vi "MotorControl.vi"() -> ()   [LabVIEW 2017]
panel:
  out "output cluster":T1={"Motor Relative"=[0.0, 0.0, 0.0, 0.0], "Motor absolute"=[0.0, 0.0, 0.0, 0.0], "Motor zero"=[0.0, 0.0, 0.0, 0.0], "Time between steps"=0.0, "Conversion (steps/mm)"=[31496.063, 31496.063, 31496.063, 12500.0], "Distance  (mm)"=[-100.0, 0.0, 0.0, 0.0], "run number"=37, "Number of steps"=1}
  in  "Module?":bool=TRUE
  in  "Stop":bool
  in  "Motor control":enum32{"Movement", "Setup", "Error"}(tab)
  in  "Single motion":bool=TRUE
  out "Step number":i32=1
  out "Motor Relative":dbl[](array[numeric])
  in  "Speed (mm/s)":dbl[](array[numeric])=[10.0, 1.0, 5.0, 10.0] format="%#_13g"
  in  "Distance  (mm)":dbl[](array[numeric])=[-100.0, 0.0, 0.0, 0.0] format="%#_13g"
  in  "Send":bool
  in  "Stop motion":bool
  out "Moving":bool
  out "Acquiring":bool
  in  "Go to zero":bool
  out "Motor Status":bool=TRUE
  out "Number of steps":i32=1
  out "Time between steps":dbl format="%#_13g"
  out "run number":i32=37
  in  "Reset motor":bool
  in  "Inc run #":bool
  in  "Zero C":bool
  in  "Zero B":bool
  in  "Zero A":bool
  in  "Zero D":bool
  in  "Motor zero":dbl[](array[numeric])=[0.0, 0.0, 0.0, 0.0] format="%#_13g"
  out "Motor absolute":dbl[](array[numeric])
  in  "Motor Port":string="COM12 19200"
  in  "Time between steps ctrl":dbl=5.0 caption="Time Target (s)"
  in  "# steps ctrl":i32=3
  in  "Conversion (steps/mm)":dbl[](array[numeric])=[31496.063, 31496.063, 31496.063, 12500.0] format="%#_13g"
  in  "Reset distance after run":bool
  in  "auto inc run #":bool
  out "error out":errorcluster={"status"=TRUE, "code"=-2147467259, "source"="Exception occured in Galil: 5001 OPEN ERROR.  OFFLINE specified to Galil::Galil()\n in MotorControl.vi"}
  out "Library Version":string="GalilClass1.dll 1.5.0.0\r\nGalil1.dll 1.6.4.580"
  out "Connect To:":string="COM12 19200, DMC2182sH2a, 16295"
  in  "Galil.IGalil":refnum<k7>
  # "spend time updating output cluster?"
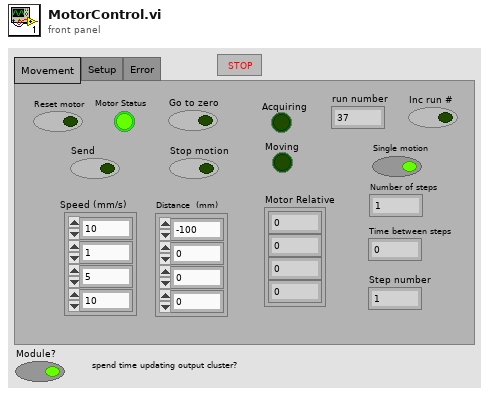
[diagram p1: front panel]
types:
  T1 = cluster{"Motor Relative":dbl[], "Motor absolute":dbl[], "Motor zero":dbl[], "Time between steps":dbl, "Conversion (steps/mm)":dbl[], "Distance  (mm)":dbl[], "run number":i32, "Number of steps":i32}
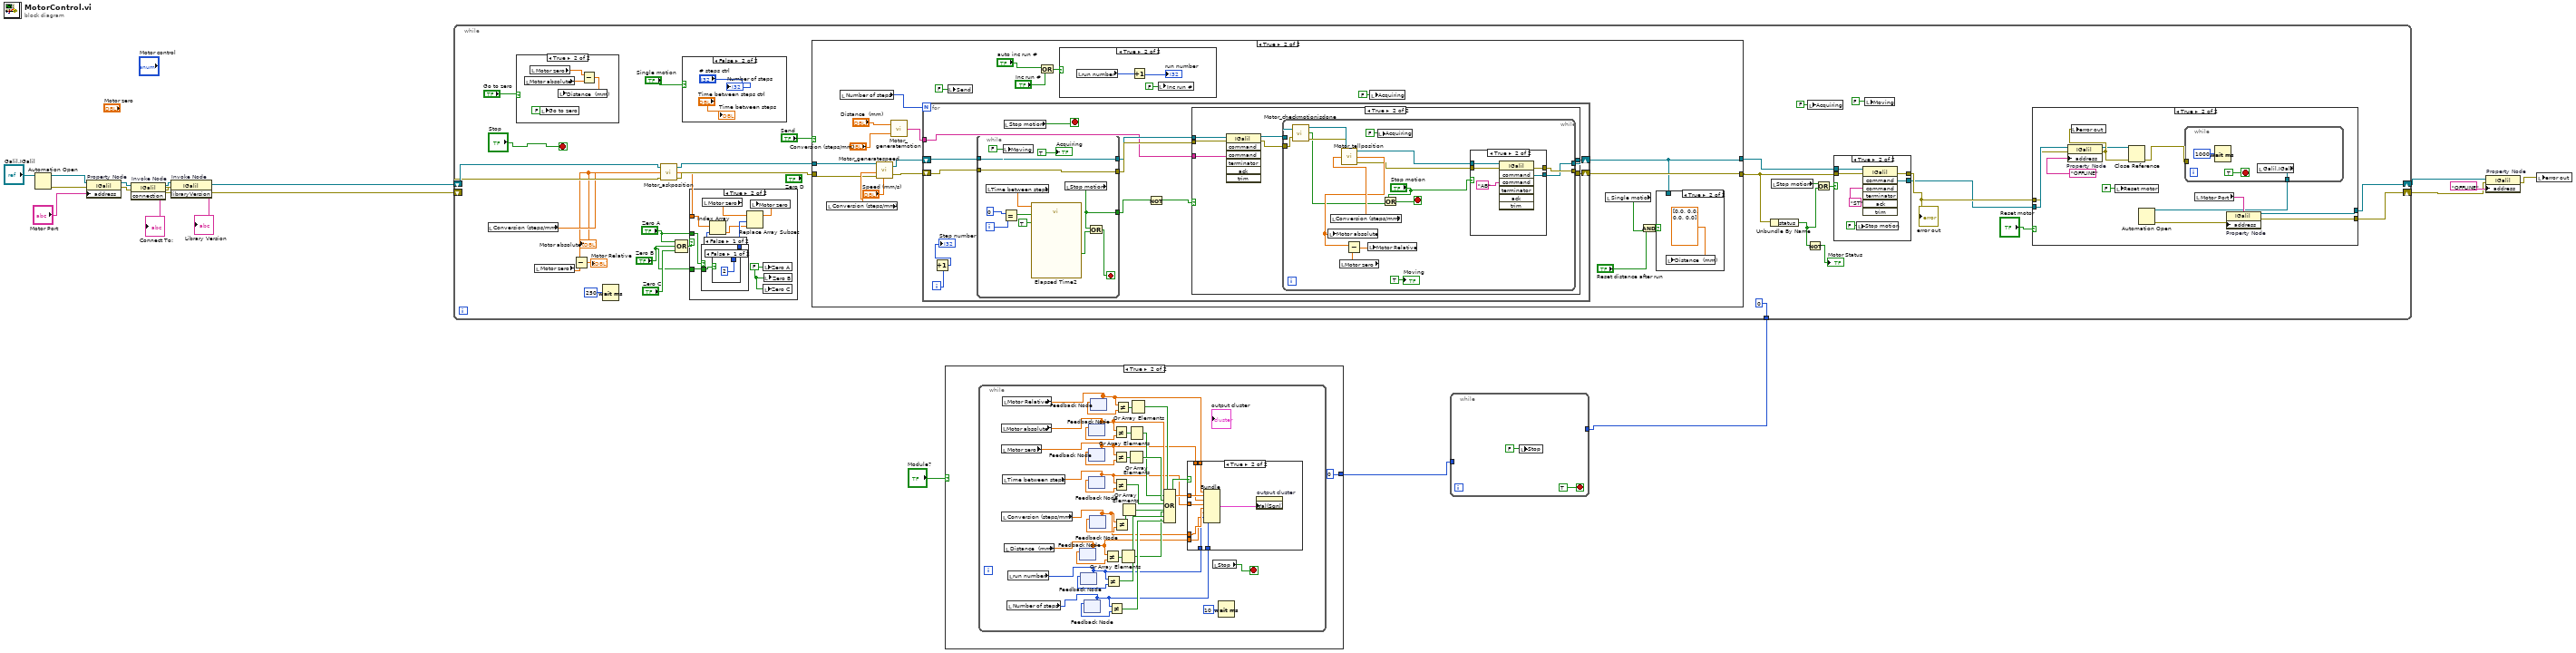
[diagram p0: block diagram]
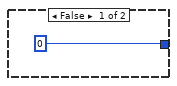
[diagram p2: hidden frame]
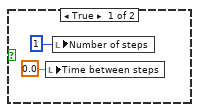
[diagram p7: hidden frame]
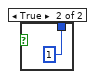
[diagram p9: hidden frame]
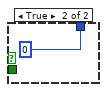
[diagram p10: hidden frame]
diagram:
  n1 = Automation Open(Automation Refnum="Galil.IGalil") -> (Automation Refnum=w13:refnum<k7>, error out=w17:errorcluster)  [unwired: 3 in]
  n2 = property on="Property Node" class="IGalil"(reference=w13, error in=w17, "address"="Motor Port") -> (reference out=w18:refnum<k7>, error out=w16:errorcluster)
  n3 = invoke on="Invoke Node" class="IGalil" method="connection"(reference=w18, error in=w16) -> (reference out=w12:refnum<k7>, error out=w11:errorcluster, "connection"=→"Connect To:":string)  [unwired: 1 in]
  n4 = invoke on="Invoke Node" class="IGalil" method="libraryVersion"(reference=w12, error in=w11) -> (reference out=w9:refnum<k7>, error out=w8:errorcluster, "libraryVersion"=→"Library Version":string)  [unwired: 1 in]
  n5 = while {
    shift-right: [w23] -> w6
    shift-left: w9 -> [w34]
    shift-right: [w22] -> w5
    shift-left: w8 -> [w33]
    tunnel: [0] -> w1
    stop <- "Stop" stop-if-true
    n6 = local read "Conversion (steps/mm)"() -> (w30:dbl[])
    n7 = case shown="True" "Go to zero" {
      frame False {
      }
      frame True {
        n8 = local read "Motor absolute"() -> (w70:dbl[])
        n9 = local read "Motor zero"() -> (w71:dbl[])
        n10 = local write "Go to zero"(FALSE ("Zero A")) -> ()
        n11 = Subtract(x=w71, y=w70) -> (x-y=w69:dbl[])
        n12 = local write "Distance  (mm)"(w69) -> ()
      }
    }
    n13 = local read "Motor zero"() -> (w46:dbl[])
    n14 = Wait (ms)(milliseconds to wait=u32 250) -> ()  [unwired: 1 out]
    n15 = call "Motor_askposition.vi"("error in (no error)"=w33, "Conversion\n (steps/mm)"=w30, "reference"=w34) -> ("error out"=w31:errorcluster, "position out"=w29:dbl[], "reference out"=w32:refnum<k7>)
    "Motor absolute" <- w29
    n16 = Subtract(x=w29, y=w46) -> (x-y=→"Motor Relative":dbl[])
    n17 = Compound Arithmetic op=OR("Zero A", "Zero B", "Zero C") -> (w37:bool)
    n18 = case shown="False" "Single motion" {
      frame True {
        n19 = local write "Time between steps"(0.0 ("Time between steps")) -> ()
        n20 = local write "Number of steps"(1 ("Number of steps")) -> ()
      }
      frame False {
        "Number of steps" <- "# steps ctrl"
        "Time between steps" <- "Time between steps ctrl"
      }
    }
    n21 = case shown="True" w37 {
      tunnel: w29 -> [_ w87]
      tunnel: "Zero A" -> [_ w90]
      tunnel: "Zero B" -> [_ w89]
      frame False {
      }
      frame True {
        w92 = FALSE ("Zero A")
        n22 = case shown="False" w90 {
          tunnel: [w93 0] -> w88
          tunnel: w89 -> [w94 _]
          frame False {
            n23 = case shown="False" w94 {
              tunnel: [2 1] -> w93
              frame False {
              }
              frame True {
              }
            }
          }
          frame True {
          }
        }
        n24 = local read "Motor zero"() -> (w91:dbl[])
        n25 = Index Array(array=w87, index=w88) -> (element=w86:dbl)
        n26 = Replace Array Subset(array=w91, new element=w86, index=w88) -> (w85:dbl[])
        n27 = local write "Motor zero"(w85) -> ()
        n28 = local write "Zero A"(w92) -> ()
        n29 = local write "Zero C"(w92) -> ()
        n30 = local write "Zero B"(w92) -> ()
      }
    }
    n31 = case shown="True" "Send" {
      tunnel: w32 -> [w99 w109]
      tunnel: w31 -> [w98 w108]
      tunnel: [w99 w110] -> w42
      tunnel: [w98 w118] -> w39
      frame False {
      }
      frame True {
        n32 = local read "Conversion (steps/mm)"() -> (w111:dbl[])
        n33 = local read "Number of steps"() -> (w116:i32)
        n34 = call "Motor_generatespeed.vi"("error in (no error)"=w108, "Conversion\n (steps/mm)"=w111, "Speed (mm/s)"="Speed (mm/s)", "reference"=w109) -> ("error out"=w106:errorcluster, "reference out"=w107:refnum<k7>)
        n35 = call "Motor_generatemotion.vi"("Conversion\n (steps/mm)"="Conversion (steps/mm)", "Distance  (mm)"="Distance  (mm)") -> ("Movement string"=w113:string)
        n36 = for {
          N: w116 -> [_]
          tunnel: w113 -> [w124]
          shift-right: [w130] -> w110
          shift-left: w107 -> [w132]
          shift-right: [w129] -> w118
          shift-left: w106 -> [w131]
          i -> [w134]
          stop <- w135 stop-if-true
          n37 = Increment(x=w134) -> (x+1=→"Step number":i32)
          n38 = while {
            tunnel: w132 -> [w179]
            tunnel: [w180] -> w126
            tunnel: w131 -> [w180]
            tunnel: [w179] -> w125
            tunnel: [w169] -> w127
            i -> [w175]
            stop <- w177 stop-if-true
            n39 = local read "Time between steps"() -> (w171:dbl)
            n40 = local write "Moving"(FALSE ("Aquiring")) -> ()
            n41 = Equal?(x=0, y=w175) -> (x = y?=w173:bool)
            n42 = call "Elapsed Time2"("Time Target (s)"=w171, "Reset"=w173, "Auto Reset"=TRUE) -> ("Time has Elapsed"=w178:bool)  [unwired: 9 in, 7 out]
            n43 = local read "Stop motion"() -> (w169:bool)
            n44 = Or(x=w169, y=w178) -> (x .or. y?=w177:bool)
            "Acquiring" <- TRUE
          }
          n45 = local read "Stop motion"() -> (w135:bool)
          n46 = Not(x=w127) -> (.not. x?=w128:bool)
          n47 = case shown="True" w128 {
            tunnel: w125 -> [w137 w142]
            tunnel: w126 -> [w136 w139]
            tunnel: [w137 w144] -> w130
            tunnel: [w136 w143] -> w129
            tunnel: w124 -> [_ w138]
            frame False {
            }
            frame True {
              n48 = invoke class="IGalil" method="command"(reference=w142, error in=w139, "command"=w138) -> (reference out=w141:refnum<k7>, error out=w140:errorcluster)  [unwired: 4 in, 5 out]
              n49 = while {
                tunnel: w141 -> [w154]
                tunnel: [w147] -> w144
                tunnel: [w148] -> w143
                tunnel: w140 -> [w145]
                stop <- w160 stop-if-true
                n50 = call "Motor_checkmotionisdone.vi"("reference"=w154, "error in (no error)"=w145) -> ("reference out"=w153:refnum<k7>, "Motion is done"=w151:bool, "error out"=w152:errorcluster)
                n51 = local read "Conversion (steps/mm)"() -> (w156:dbl[])
                n52 = local read "Motor zero"() -> (w159:dbl[])
                n53 = call "Motor_tellposition.vi"("error in (no error)"=w152, "Conversion\n (steps/mm)"=w156, "reference"=w153) -> ("error out"=w149:errorcluster, "Position out"=w155:dbl[], "reference out"=w150:refnum<k7>)
                n54 = local write "Motor absolute"(w155) -> ()
                n55 = Subtract(x=w155, y=w159) -> (x-y=w158:dbl[])
                n56 = local write "Motor Relative"(w158) -> ()
                n57 = local write "Acquiring"(FALSE ("Aquiring")) -> ()
                n58 = Or(x="Stop motion", y=w151) -> (x .or. y?=w160:bool)
                n59 = case shown="True" "Stop motion" {
                  tunnel: w150 -> [w163 w167]
                  tunnel: w149 -> [w162 w166]
                  tunnel: [w163 w165] -> w147
                  tunnel: [w162 w164] -> w148
                  frame False {
                  }
                  frame True {
                    n60 = invoke class="IGalil" method="command"(reference=w167, error in=w166, "command"="AB") -> (reference out=w165:refnum<k7>, error out=w164:errorcluster)  [unwired: 4 in, 5 out]
                  }
                }
                "Moving" <- TRUE
              }
            }
          }
        }
        n61 = local write "Send"(FALSE ("Send")) -> ()
        n62 = Or(x="auto inc run #", y="Inc run #") -> (x .or. y?=w102:bool)
        n63 = case shown="True" w102 {
          frame False {
          }
          frame True {
            n64 = local read "run number"() -> (w121:i32)
            n65 = Increment(x=w121) -> (x+1=→"run number":i32)
            n66 = local write "Inc run #"(FALSE ("Inc run #")) -> ()
          }
        }
        n67 = local write "Acquiring"(FALSE ("Aquiring")) -> ()
        n68 = local read "Single motion"() -> (w104:bool)
        n69 = And(x="Reset distance after run", y=w104) -> (x .and. y?=w105:bool)
        n70 = case shown="True" w105 {
          tunnel: w110 -> [_ _]
          frame False {
          }
          frame True {
            n71 = local write "Distance  (mm)"(dbl[] [0.0, 0.0, 0.0, 0.0] ("Distance  (mm)")) -> ()
          }
        }
      }
    }
    n72 = Unbundle By Name(w39) -> ("status"=w27:bool)
    n73 = local read "Stop motion"() -> (w40:bool)
    n74 = Not(x=w27) -> (.not. x?=→"Motor Status":bool)
    n75 = local write "Acquiring"(FALSE ("Aquiring")) -> ()
    n76 = Or(x=w40, y=w27) -> (x .or. y?=w41:bool)
    n77 = case shown="True" w41 {
      tunnel: w42 -> [w74 w79]
      tunnel: w39 -> [w73 w78]
      tunnel: [w74 w77] -> w24
      tunnel: [w73 w76] -> w25
      frame False {
      }
      frame True {
        n78 = local write "Stop motion"(FALSE ("Stop motion")) -> ()
        n79 = invoke class="IGalil" method="command"(reference=w79, error in=w78, "command"="ST") -> (reference out=w77:refnum<k7>, error out=w76:errorcluster)  [unwired: 4 in, 5 out]
      }
    }
    "error out" <- w25
    n80 = local write "Moving"(FALSE ("Waiting")) -> ()
    n81 = case shown="True" "Reset motor" {
      tunnel: w24 -> [w51 w54]
      tunnel: w25 -> [w52 w53]
      tunnel: [w51 w64] -> w23
      tunnel: [w52 w65] -> w22
      frame False {
      }
      frame True {
        n82 = property on="Property Node" class="IGalil"(reference=w54, error in=w53, "address"="OFFLINE") -> (reference out=w57:refnum<k7>, error out=w58:errorcluster)
        n83 = local write "error out"(w58) -> ()
        n84 = local write "Reset motor"(FALSE ("Reset motor")) -> ()
        n85 = Close Reference(reference=w57, error in (no error)=w58) -> (error out=w55:errorcluster)
        n86 = while {
          tunnel: [w66] -> w62
          tunnel: w55 -> [_]
          stop <- TRUE stop-if-true
          n87 = Wait (ms)(milliseconds to wait=u32 1000) -> ()  [unwired: 1 out]
          n88 = local read "Galil.IGalil"() -> (w66:refnum<k7>)
        }
        n89 = Automation Open(Automation Refnum=w62) -> (Automation Refnum=w61:refnum<k7>, error out=w60:errorcluster)  [unwired: 3 in]
        n90 = local read "Motor Port"() -> (w63:string)
        n91 = property on="Property Node" class="IGalil"(reference=w61, error in=w60, "address"=w63) -> (reference out=w64:refnum<k7>, error out=w65:errorcluster)
      }
    }
  }
  n92 = case shown="True" "Module?" {
    tunnel: [0 0] -> w2
    frame False {
    }
    frame True {
      n93 = while {
        stop <- w214 stop-if-true
        n94 = local read "Motor absolute"() -> (w200:dbl[])
        n95 = local read "Motor zero"() -> (w188:dbl[])
        n96 = local read "Conversion (steps/mm)"() -> (w186:dbl[])
        n97 = local read "Motor Relative"() -> (w201:dbl[])
        n98 = local read "Time between steps"() -> (w187:dbl)
        n99 = local read "Distance  (mm)"() -> (w185:dbl[])
        n100 = local read "Number of steps"() -> (w183:i32)
        n101 = local read "run number"() -> (w184:i32)
        n102 = feedback #1() -> (w207:dbl[])  [unwired: 1 in]
        n103 = feedback-in #1(w185) -> ()
        n104 = feedback #2() -> (w206:i32)  [unwired: 1 in]
        n105 = feedback-in #2(w184) -> ()
        n106 = feedback #3() -> (w205:i32)  [unwired: 1 in]
        n107 = feedback-in #3(w183) -> ()
        n108 = feedback #4() -> (w211:dbl[])  [unwired: 1 in]
        n109 = feedback-in #4(w200) -> ()
        n110 = feedback #5() -> (w210:dbl[])  [unwired: 1 in]
        n111 = feedback-in #5(w188) -> ()
        n112 = feedback #6() -> (w209:dbl)  [unwired: 1 in]
        n113 = feedback-in #6(w187) -> ()
        n114 = feedback #7() -> (w208:dbl[])  [unwired: 1 in]
        n115 = feedback-in #7(w186) -> ()
        n116 = feedback-in #8(w201) -> ()
        n117 = feedback #8() -> (w212:dbl[])  [unwired: 1 in]
        n118 = Not Equal?(x=w185, y=w207) -> (x != y?=w199:bool[])
        n119 = Not Equal?(x=w184, y=w206) -> (x != y?=w203:bool)
        n120 = Not Equal?(x=w183, y=w205) -> (x != y?=w202:bool)
        n121 = Not Equal?(x=w200, y=w211) -> (x != y?=w197:bool[])
        n122 = Not Equal?(x=w188, y=w210) -> (x != y?=w195:bool[])
        n123 = Not Equal?(x=w187, y=w209) -> (x != y?=w204:bool)
        n124 = Not Equal?(x=w186, y=w208) -> (x != y?=w198:bool[])
        n125 = Not Equal?(x=w201, y=w212) -> (x != y?=w196:bool[])
        n126 = Or Array Elements(Boolean array=w199) -> (logical OR=w190:bool)
        n127 = Or Array Elements(Boolean array=w198) -> (logical OR=w191:bool)
        n128 = Or Array Elements(Boolean array=w195) -> (logical OR=w194:bool)
        n129 = Or Array Elements(Boolean array=w197) -> (logical OR=w193:bool)
        n130 = Or Array Elements(Boolean array=w196) -> (logical OR=w192:bool)
        n131 = Compound Arithmetic op=OR(w192, w193, w194, w204, w191, w190, w203, w202) -> (w189:bool)
        n132 = case shown="True" w189 {
          tunnel: w201 -> [_ w223]
          tunnel: w200 -> [_ w222]
          tunnel: w188 -> [_ w221]
          tunnel: w187 -> [_ w220]
          tunnel: w186 -> [_ w219]
          tunnel: w185 -> [_ w218]
          tunnel: w184 -> [_ w217]
          tunnel: w183 -> [_ w216]
          frame False {
          }
          frame True {
            n133 = Bundle("Motor Relative"=w223, "Motor absolute"=w222, "Motor zero"=w221, "Time between steps"=w220, "Conversion (steps/mm)"=w219, "Distance  (mm)"=w218, "run number"=w217, "Number of steps"=w216) -> (w215:T1)  [unwired: 1 in]
            n134 = property on="output cluster" class="Clust (strict)"("Val(Sgnl)"=w215) -> ()  [unwired: 2 in, 2 out]
          }
        }
        n135 = local read "Stop"() -> (w214:bool)
        n136 = Wait (ms)(milliseconds to wait=u32 10) -> ()  [unwired: 1 out]
      }
    }
  }
  n137 = while {
    tunnel: w2 -> [_]
    tunnel: w1 -> [_]
    stop <- TRUE stop-if-true
    n138 = local write "Stop"(FALSE ("stop")) -> ()
  }
  n139 = property on="Property Node" class="IGalil"(reference=w6, error in=w5, "address"="OFFLINE") -> (error out=w4:errorcluster)  [unwired: 1 out]
  n140 = local write "error out"(w4) -> ()
